vi "CLD3 FGV Timer Exercise.vi"(8 "Error In":errorcluster, 10 "Time Target (s)":dbl=4.0, 11 "Timer Mode":T1) -> (0 "Error Out":errorcluster, 3 "Elapsed Time (s.ss)":dbl)   [LabVIEW 2018]
doc: "CLD 3 Exercise"
uses:
  CLD3 FGV Mode.ctl
panel:
  in  "Stop Button":bool
  out "Has Time Elapsed":bool
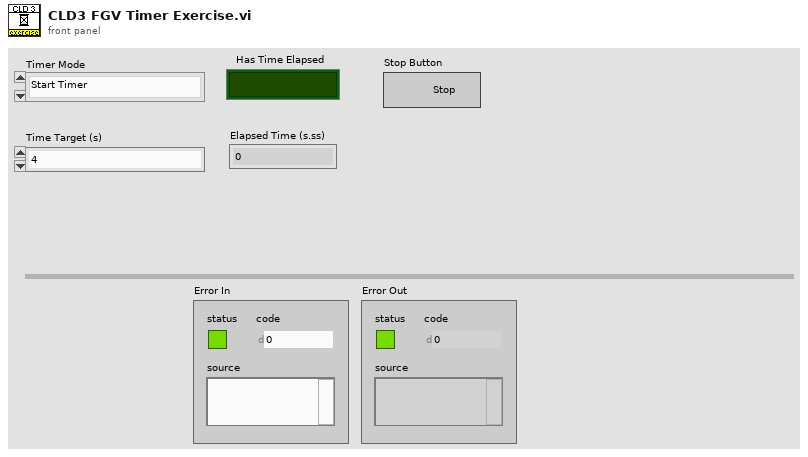
[diagram p1: front panel]
types:
  T1 = typedef "CLD3 FGV Mode.ctl" = enum16{"Start Timer", "Read Time", "Pause", "Resume"}
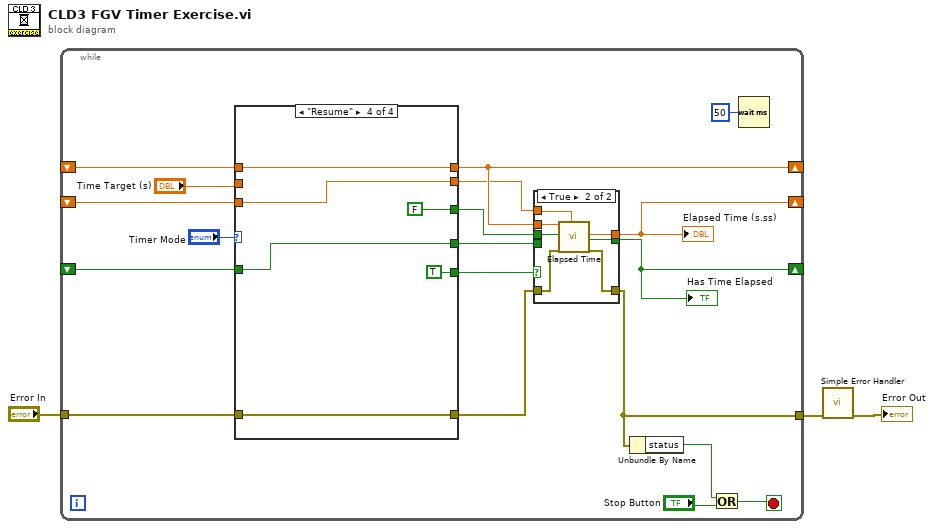
[diagram p0: block diagram]
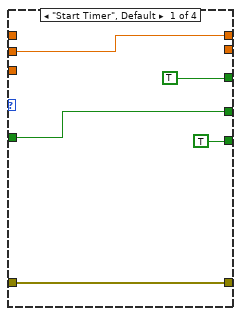
[diagram p3: hidden frame]
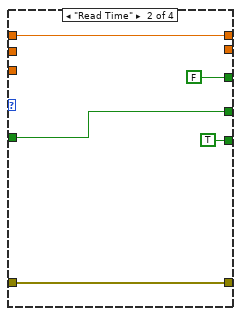
[diagram p4: hidden frame]
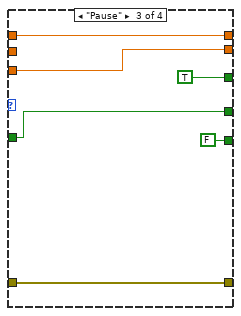
[diagram p5: hidden frame]
diagram:
  n1 = while {
    tunnel: "Error In" -> [w18]
    tunnel: [w10] -> w2
    shift-right: [w17] -> _
    shift-left: _ -> [w21]
    shift-right: [w16] -> _
    shift-left: _ -> [w15]
    shift-right: [w14] -> _
    shift-left: _ -> [w13]
    stop <- w9 stop-if-true
    n2 = case shown="\"Resume\"" "Timer Mode" {
      tunnel: w21 -> [_ w42 w46 w53]
      tunnel: [w35 w42 w46 w53] -> w17
      tunnel: [TRUE FALSE TRUE FALSE] -> w20
      tunnel: [w36 w40 w45 w51] -> w19
      tunnel: w18 -> [w36 w40 w45 w51]
      tunnel: "Time Target (s)" -> [w35 _ _ _]
      tunnel: w15 -> [w33 w38 w44 w50]
      tunnel: w13 -> [_ _ w47 w54]
      tunnel: [_ _ w47 w54] -> w12
      tunnel: [TRUE TRUE FALSE TRUE] -> w6
      tunnel: [w33 w38 w44 w50] -> w5
      frame "Start Timer", Default {
      }
      frame "Read Time" {
      }
      frame "Pause" {
      }
      frame "Resume" {
      }
    }
    n3 = case shown="True" w6 {
      tunnel: w20 -> [_ w32]
      tunnel: w19 -> [w24 w31]
      tunnel: w17 -> [_ w30]
      tunnel: [w23 w29] -> w16
      tunnel: [w25 w28] -> w14
      tunnel: w12 -> [w25 w27]
      tunnel: [w24 w26] -> w10
      tunnel: w5 -> [w23 _]
      frame False {
      }
      frame True {
        n4 = call "Elapsed Time"("Time Target (s)"=w30, "Reset"=w32, "error in (no error)"=w31, "Set Start Time (s)"=w27) -> ("Elapsed Time (s)"=w28:dbl, "Time has Elapsed"=w29:bool, "error out"=w26:errorcluster)  [unwired: 8 in, 5 out]
      }
    }
    "Has Time Elapsed" <- w16
    "Elapsed Time (s.ss)" <- w14
    n5 = Unbundle By Name(w10) -> ("status"=w7:bool)
    n6 = Or(x=w7, y="Stop Button") -> (x .or. y?=w9:bool)
    n7 = Wait (ms)(milliseconds to wait=u32 50) -> ()  [unwired: 1 out]
  }
  n8 = call <vilib>:"Simple Error Handler.vi"("error in (no error)"=w2) -> ("error out"=→"Error Out":errorcluster)  [unwired: 4 in, 4 out]
